vi "Encode JSON.vi"(4 "error in (no error)":errorcluster, 7 "JSON Tree In":variant) -> (0 "error out":errorcluster, 2 "String":string)   [LabVIEW 2013, in "i3-json.lvlib"]
doc: "Flattens a JSON Tree to a JSON String"
uses:
  i3-json.lvlib
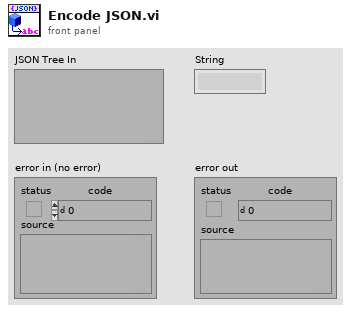
[diagram p1: front panel]
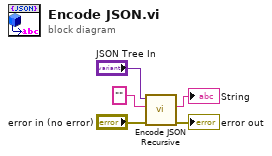
[diagram p0: block diagram]
diagram:
  n1 = call "Encode JSON Recursive.vi"("error in (no error)"="error in (no error)", "String In"="", "JSON Tree"="JSON Tree In") -> ("error out"=→"error out":errorcluster, "String Out"=→"String":string)  [unwired: 3 in]
